vi "isExcluded.vi"(8 "error in (no error)":errorcluster, 11 "Outcome in":refnum<class "Outcome.lvclass">) -> (0 "error out":errorcluster, 2 "Excluded?":bool, 3 "Outcome out":refnum<class "Outcome.lvclass">)   [LabVIEW 2018, in "Outcome.lvclass"]
uses:
  Outcome.lvclass
  Outcome.lvclass/Outcome.ctl
  Goal/Goal.lvclass
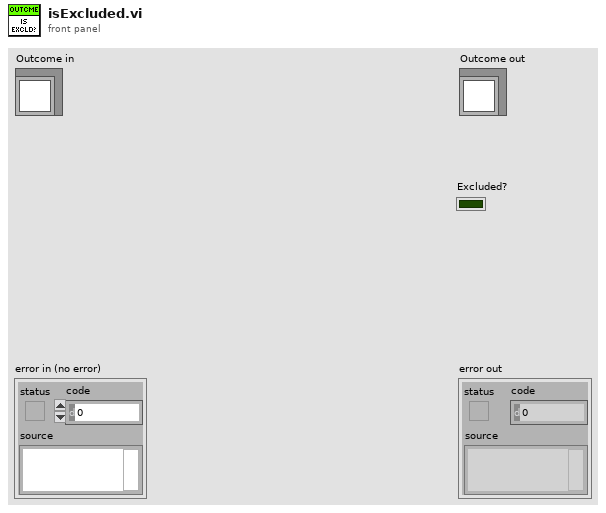
[diagram p1: front panel]
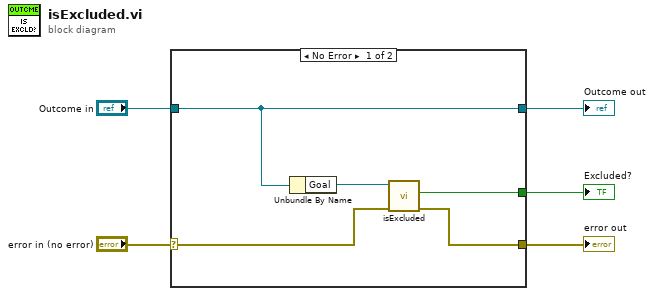
[diagram p0: block diagram]
diagram:
  n1 = case shown="No Error" "error in (no error)" {
    selector: "error in (no error)" -> [w8 w12]
    tunnel: [w7 w12] -> w4
    tunnel: [w10 w11] -> w2
    tunnel: "Outcome in" -> [w10 w11]
    tunnel: [w6 _] -> w1
    frame No Error {
      n2 = Unbundle By Name(w10) -> ("Goal"=w9:refnum<class "Goal.lvclass">)
      n3 = call "isExcluded.vi"("error in (no error)"=w8, "Goal in"=w9) -> ("error out"=w7:errorcluster, "Excluded?"=w6:bool)  [unwired: 7 in, 1 out]
    }
    frame Error {
    }
  }
  "error out" <- w4
  "Outcome out" <- w2
  "Excluded?" <- w1
